vi "Create file name.vi"(8 "error in (no error)":errorcluster, 11 "Tomo in":refnum<class "Tomo.lvclass">) -> (0 "error out":errorcluster, 2 "filename":string, 3 "Tomo out":refnum<class "Tomo.lvclass">)   [LabVIEW 2012, in "Tomo.lvclass"]
uses:
  Tomo.lvclass
  Tomo.lvclass/Tomo.ctl
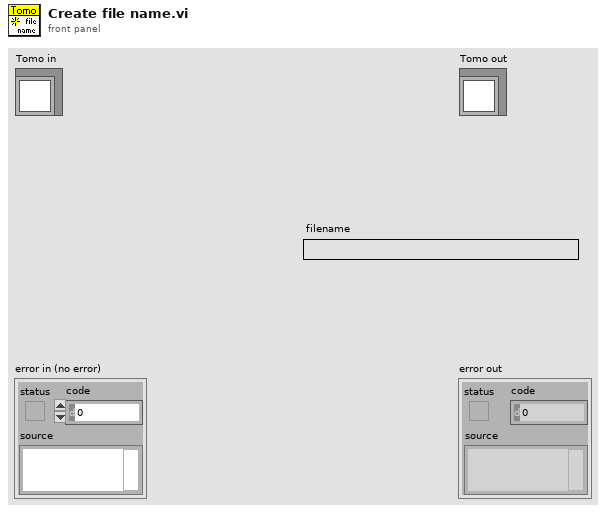
[diagram p1: front panel]
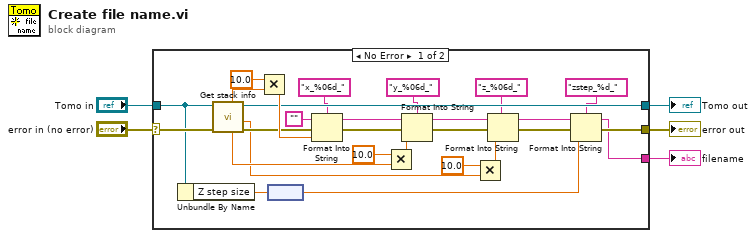
[diagram p0: block diagram]
diagram:
  n1 = case shown="No Error" "error in (no error)" {
    selector: "error in (no error)" -> [w33 w35]
    tunnel: [w7 w35] -> w4
    tunnel: [w15 w34] -> w2
    tunnel: "Tomo in" -> [w14 w34]
    tunnel: [w6 _] -> w1
    frame No Error {
      n2 = Unbundle By Name(w14) -> ("Z step size"=w13:dbl[unit])
      n3 = call-dynamic "Get stack info.vi"("error in (no error)"=w33, "Tomo in"=w14) -> ("error out"=w29:errorcluster, "Z start"=w17:dbl, "Tomo out"=w15:refnum<class "Tomo.lvclass">, "Y position"=w19:dbl, "X position"=w31:dbl)  [unwired: 4 in, 1 out]
      n4 = Multiply(x=10.0, y=w31) -> (x*y=w32:dbl)
      n5 = node(w13) -> (w12:dbl)
      n6 = Format Into String(format string="x_%06d_", initial string="", error in=w29, w32) -> (resulting string=w22:string, error out=w28:errorcluster)
      n7 = Multiply(x=10.0, y=w19) -> (x*y=w18:dbl)
      n8 = Format Into String(format string="y_%06d_", initial string=w22, error in=w28, w18) -> (resulting string=w21:string, error out=w27:errorcluster)
      n9 = Multiply(x=10.0, y=w17) -> (x*y=w16:dbl)
      n10 = Format Into String(format string="z_%06d_", initial string=w21, error in=w27, w16) -> (resulting string=w20:string, error out=w26:errorcluster)
      n11 = Format Into String(format string="zstep_%d_", initial string=w20, error in=w26, w12) -> (resulting string=w6:string, error out=w7:errorcluster)
    }
    frame Error {
    }
  }
  "error out" <- w4
  "Tomo out" <- w2
  "filename" <- w1
